vi "ROS_Master_AddService.vi"(2 "String w/o Tag":string, 3 "ROS_Master in":T1) -> (0 "Service":T4, 1 "ROS_Master out":T1)   [LabVIEW 2012]
doc: "Registers a service with the master"
uses:
  <userlib>/ROS for LabVIEW Software/ROS/Code/ROS_Master/ROS_Service.ctl
  <userlib>/ROS for LabVIEW Software/ROS/Code/ROS_Master/ROS_Master.ctl
  <userlib>/ROS for LabVIEW Software/ROS/Code/ROS_Master/ROS_Topic.ctl
  <userlib>/ROS for LabVIEW Software/ROS/Code/ROS_Master/ROS_Node.ctl
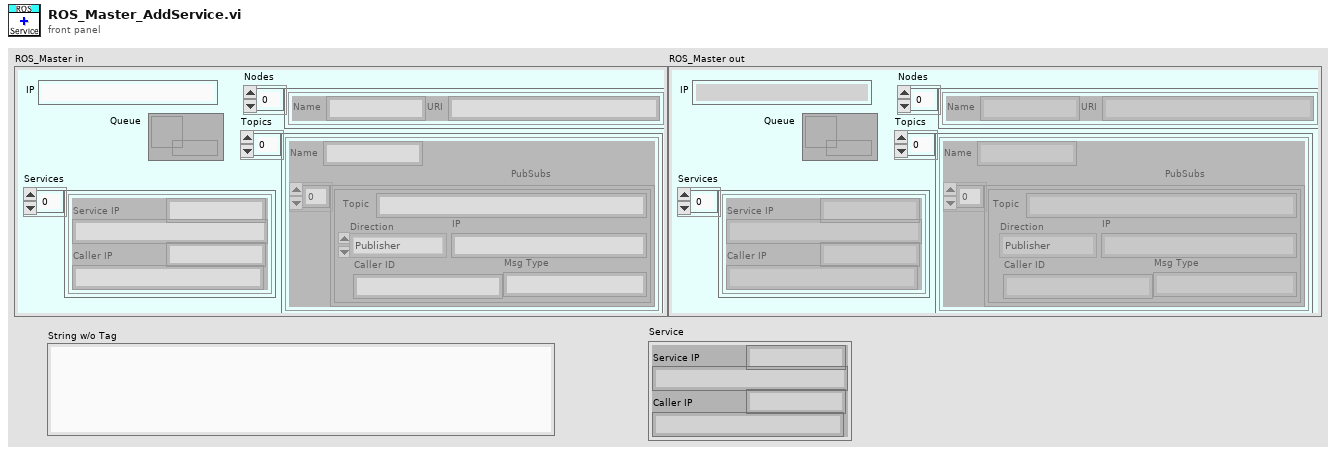
[diagram p1: front panel]
types:
  T1 = typedef "ROS_Master.ctl" = cluster{"IP":string, "Topics":cluster{"Name":string, "PubSubs":T2[]}[], "Nodes":T3[], "Services":T4[], "Queue":refnum<queue>}
  T2 = typedef "ROS_Topic.ctl" = cluster{"Caller ID":string, "IP":string, "Msg Type":string, "Direction":enum16{"Publisher", "Subscriber"}, "Topic":string}
  T3 = typedef "ROS_Node.ctl" = cluster{"Name":string, "URI":string}
  T4 = typedef "ROS_Service.ctl" = cluster{"Service":string, "Service IP":string, "Caller IP":string, "Caller ID":string}
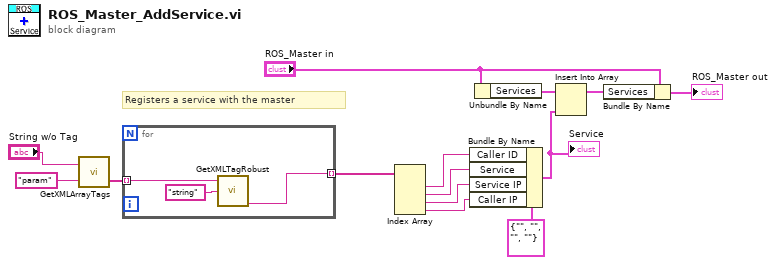
[diagram p0: block diagram]
diagram:
  # "Registers a service with the master"
  n1 = call <userlib>:"GetXMLArrayTags.vi"("ArrayTag"="param", "String"="String w/o Tag") -> ("Array"=w3:string[])  [unwired: 1 out]
  n2 = for {
    tunnel: w3 -> [w17] mode=indexing
    tunnel: [w15] -> w4 mode=indexing
    n3 = call <userlib>:"GetXMLTagRobust.vi"("Tag"="string", "String"=w17) -> ("value"=w15:string)  [unwired: 1 in, 3 out]
  }
  n4 = Index Array(array=w4) -> (element #1=w6:string, element #2=w7:string, element #3=w8:string, element #4=w11:string)  [unwired: 4 in]
  n5 = Bundle By Name(cluster=T4 {"Service"="", "Service IP"="", "Caller IP"="", "Caller ID"=""} ("Service"), "Caller ID"=w6, "Service"=w7, "Service IP"=w8, "Caller IP"=w11) -> (w13:T4)
  "Service" <- w13
  n6 = Unbundle By Name("ROS_Master in") -> ("Services"=w9:T4[])
  n7 = Insert Into Array(array=w9, new element=w13) -> (w12:T4[])  [unwired: 1 in]
  n8 = Bundle By Name(cluster="ROS_Master in", "Services"=w12) -> (→"ROS_Master out":T1)
